vi "Averager Compute.vi"(8 "error in (no error)":errorcluster, 10 "Data":dbl[](array[numeric]), 11 "Averager in":refnum<class "Averager.lvclass">) -> (0 "error out":errorcluster, 3 "Averager out":refnum<class "Averager.lvclass">)   [LabVIEW 2018, in "Averager.lvclass"]
uses:
  Averager.lvclass
  Averager.lvclass/Averager.ctl
  <vilib>/Analysis/baseanly.llb/Mean (DBL).vi
  <vilib>/Analysis/NI_AALBase.lvlib
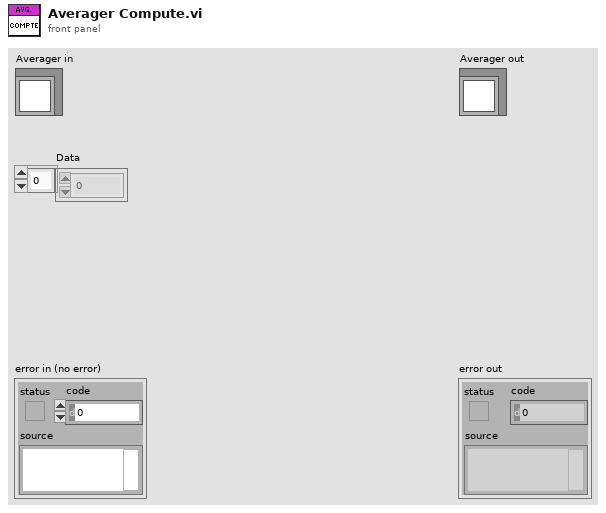
[diagram p1: front panel]
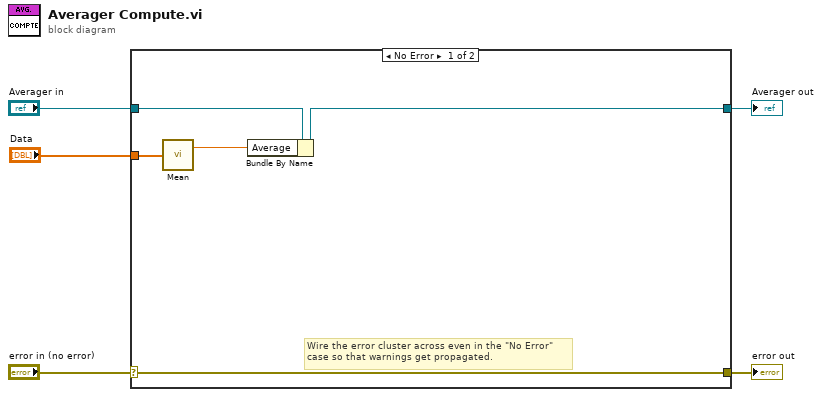
[diagram p0: block diagram]
diagram:
  n1 = case shown="No Error" "error in (no error)" {
    selector: "error in (no error)" -> [w10 w12]
    tunnel: [w10 w12] -> w4
    tunnel: [w6 w11] -> w2
    tunnel: "Averager in" -> [w8 w11]
    tunnel: "Data" -> [w9 _]
    frame No Error {
      # "Wire the error cluster across even in the \"No Error\"\ncase so that warnings get propagated."
      n2 = call-poly <vilib>:"Mean.vi"("X"=w9) -> ("mean"=w7:dbl)  [unwired: 1 out]
      n3 = Bundle By Name(cluster=w8, "Average"=w7) -> (w6:refnum<class "Averager.lvclass">)
    }
    frame Error {
    }
  }
  "error out" <- w4
  "Averager out" <- w2
